vi "Read Scheduled.vi"(1 "scheduled time":timestamp, 2 "channel":T1) -> (5 "actual time":timestamp, 7 "element":string, 8 "missed":i32)   [LabVIEW 2020, in "Tag-str.lvlib"]
doc: "Reads a value from a Tag channel at a scheduled time."
uses:
  <extravilib>/ChannelInstances/Tag-str.lvlib
  <extravilib>/ChannelInstances/Tag-str/))Channel.ctl
  <extravilib>/ChannelInstances/Tag-str/Read With Abort.vi
  <extravilib>/ChannelInstances/Tag-str/EndpointRead.vi
  <resource>/ChannelSupport/_ChannelSupport/_ChannelSupport.lvlib
  <resource>/ChannelSupport/_ChannelSupport/GetErrors/FpgaChannelWireNotSupported.xnode
panel:
  # "number of values missed\n(-1 means element is stale)"
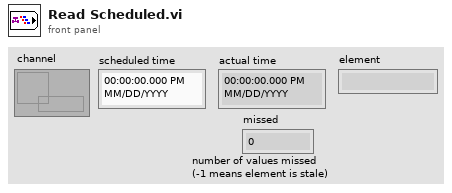
[diagram p1: front panel]
types:
  T1 = typedef "Tag-str.lvlib/))Channel.ctl" = refnum<queue>
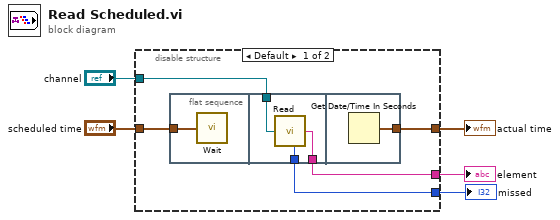
[diagram p0: block diagram]
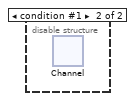
[diagram p2: hidden frame]
diagram:
  n1 = disable-structure shown="Default" {
    disable-tunnel: "scheduled time" -> [w10 _]
    disable-tunnel: [w9 _] -> w4
    disable-tunnel: "channel" -> [w8 _]
    disable-tunnel: [w7 _] -> w2
    disable-tunnel: [w6 _] -> w1
    frame condition #0 (active) {
      n2 = flat-sequence {
        tunnel: w10 -> [w11]
        tunnel: w8 -> [w14]
        tunnel: [w13] -> w7
        tunnel: [w12] -> w6
        tunnel: [w15] -> w9
        frame #0 {
          n3 = call <resource>:"Wait.vi"("desired time"=w11) -> ()  [unwired: 2 out]
        }
        frame #1 {
          n4 = call <extravilib>:"Read.vi"("channel"=w14) -> ("missed"=w12:i32, "element"=w13:string)  [unwired: 1 in]
        }
        frame #2 {
          n5 = Get Date/Time In Seconds() -> (seconds since 1Jan1904=w15:timestamp)
        }
      }
    }
    frame condition #1 {
      n6 = xnode "Channel"() -> ()
    }
  }
  "element" <- w2
  "actual time" <- w4
  "missed" <- w1
